vi "Write Cap Registers.vi"(10 "Cap Registers":T1[](array[typedef]), 11 "Toggle 6 in":refnum<class "Toggle 6.lvclass">) -> (3 "Toggle 6 out":refnum<class "Toggle 6.lvclass">)   [LabVIEW 2020, in "Toggle 6.lvclass"]
uses:
  Toggle 6.lvclass
  Controls/Capacitor register.ctl
  Toggle 6.lvclass/Toggle 6.ctl
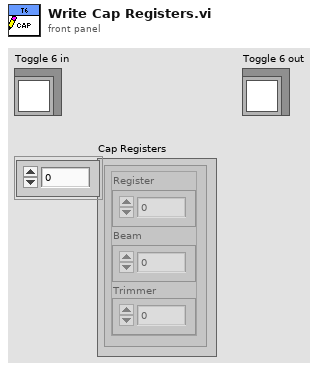
[diagram p1: front panel]
types:
  T1 = typedef "Toggle 6.lvclass/Capacitor register.ctl" = cluster{"Register":u32, "Beam":dbl, "Trimmer":dbl}
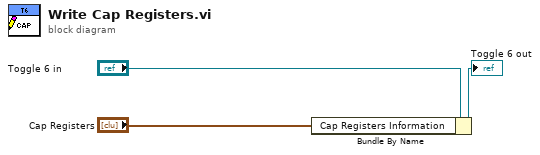
[diagram p0: block diagram]
diagram:
  n1 = Bundle By Name(cluster="Toggle 6 in", "Cap Registers Information"="Cap Registers") -> (→"Toggle 6 out":refnum<class "Toggle 6.lvclass">)
